vi "recunoastere_interfete_v2.vi"() -> (0 "Oscilloscope":string[](array[string]), 1 "DMM":string[](array[string]), 2 "Electronic Load":string[](array[string]), 3 "Source":string[](array[string]), 4 "Climate Chamber":string[](array[string]))   [LabVIEW 2022 SP3]
uses:
  <vilib>/regexp/Match Regular Expression.xnode
panel:
  out "Climate Chamber":i32
  out "Osciloscope":i32
  out "EL":i32
  out "DMM":i32
  out "Source":i32
  out "Aparatura":string[](array[string])=["TOELLNER", "AGILENT", "B&K", "LECROY", "VOTSCH"]
  out "error out":errorcluster
  in  "Instruments":string[](array[string])
  out "find list":string[](array[string])
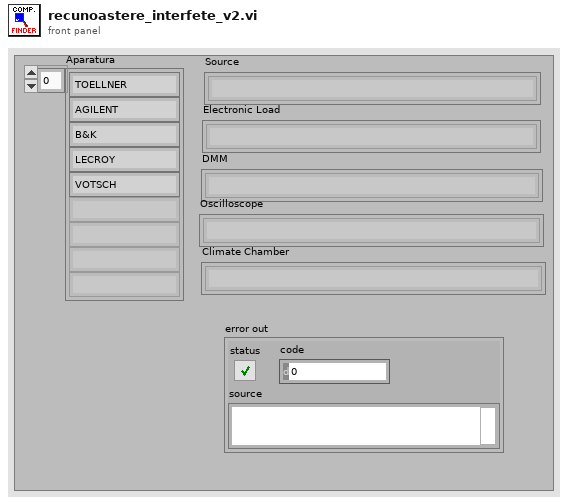
[diagram p1: front panel]
types:
  T1 = cluster{"Interface":u16, i32, "GPIB Device":u8, "GPIB Board":u8, "Direct Interface":bool, "String":string}
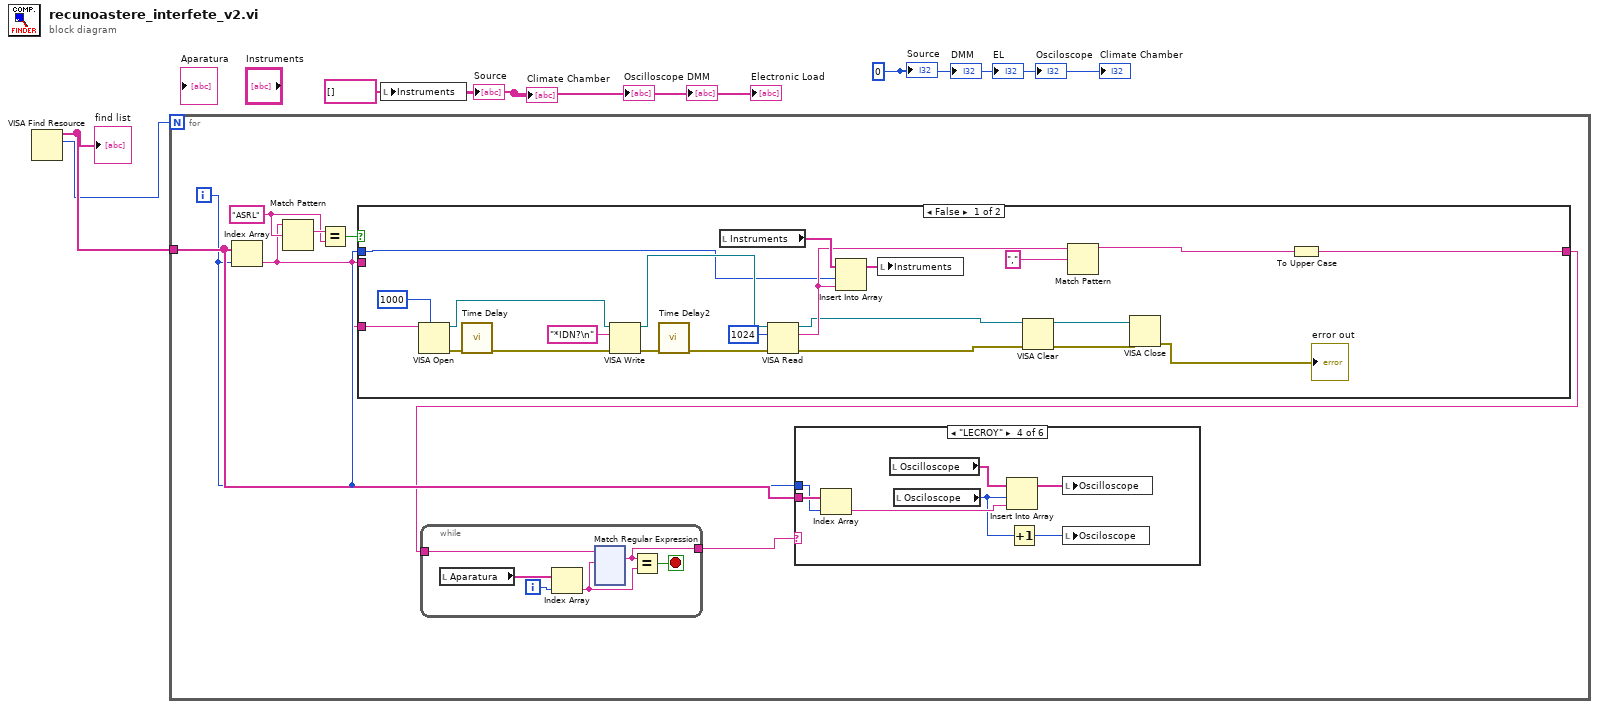
[diagram p0: block diagram]
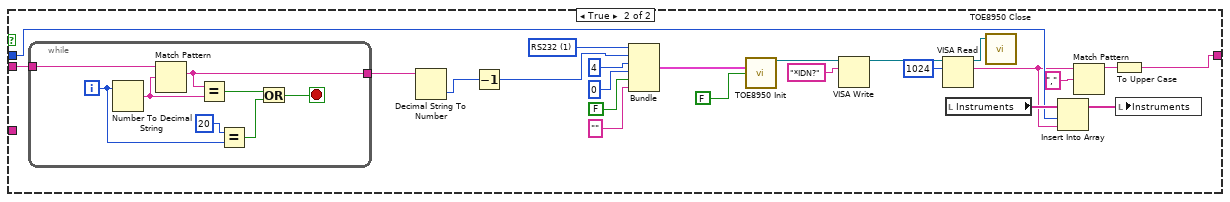
[diagram p2: hidden frame]
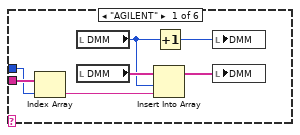
[diagram p3: hidden frame]
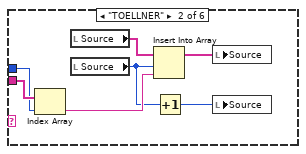
[diagram p4: hidden frame]
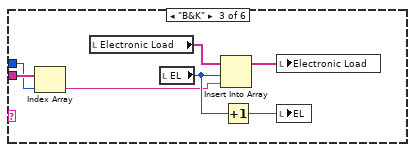
[diagram p5: hidden frame]
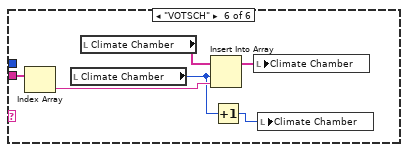
[diagram p7: hidden frame]
diagram:
  w3 = 0 ("Numeric")
  w4 = string[] [] ("Array")
  n1 = VISA Find Resource() -> (2:w1:u32, 3:w2:string[])  [unwired: 3 in, 1 out]
  "find list" <- w2
  n2 = for {
    N: w1 -> [_]
    tunnel: w2 -> [w12]
    i -> [w9]
    w7 = "ASRL" ("regular expression")
    n3 = Index Array(array=w12, index=w9) -> (element=w5:string)
    n4 = Match Pattern(string=w5, regular expression=w7) -> (match substring=w8:string)  [unwired: 1 in, 3 out]
    n5 = Equal?(x=w8, y=w7) -> (x = y?=w6:bool)
    n6 = case shown="False" w6 {
      tunnel: [w21 w39] -> w11
      tunnel: w9 -> [w20 w44]
      tunnel: w5 -> [w19 _]
      tunnel: w5 -> [_ w57]
      frame False {
        n7 = VISA Open(timeout (0)=u32 1000 ("VISA Open timeout (0)"), VISA resource name=w19) -> (VISA resource name=w29:refnum<visa-resource-name>, error out=w27:errorcluster)  [unwired: 3 in]
        n8 = call "Time Delay"("error in (no error)"=w27) -> ("error out"=w28:errorcluster)  [unwired: 10 in]
        n9 = VISA Write(VISA resource name=w29, write buffer="*IDN?\n", error in (no error)=w28) -> (VISA resource name out=w30:refnum<visa-resource-name>, error out=w26:errorcluster)  [unwired: 1 out]
        n10 = call "Time Delay2"("error in (no error)"=w26) -> ("error out"=w25:errorcluster)  [unwired: 10 in]
        n11 = local read "Instruments"() -> (w32:string[])
        n12 = VISA Read(VISA resource name=w30, byte count=u32 1024, error in (no error)=w25) -> (VISA resource name out=w17:refnum<visa-resource-name>, read buffer=w24:string, error out=w16:errorcluster)  [unwired: 1 out]
        n13 = Insert Into Array(array=w32, index=w20, new element=w24) -> (w31:string[])
        n14 = local write "Instruments"(w31) -> ()
        n15 = VISA Clear(VISA resource name=w17, error in (no error)=w16) -> (VISA resource name out=w14:refnum<visa-resource-name>, error out=w15:errorcluster)
        n16 = Match Pattern(string=w24, regular expression=",") -> (before substring=w22:string)  [unwired: 1 in, 3 out]
        n17 = VISA Close(VISA resource name=w14, error in (no error)=w15) -> (error out=→"error out":errorcluster)
        n18 = To Upper Case(1:w22) -> (0:w21:string)
      }
      frame True {
        w55 = u16 1 items=["GPIB", "RS232"] ("Interface")
        n19 = while {
          tunnel: w57 -> [w65]
          tunnel: [w58] -> w56
          i -> [w62]
          stop <- w59 stop-if-true
          n20 = Number To Decimal String(number=w62) -> (decimal integer string=w64:string)  [unwired: 1 in]
          n21 = Match Pattern(string=w65, regular expression=w64) -> (match substring=w58:string)  [unwired: 1 in, 3 out]
          n22 = Equal?(x=w58, y=w64) -> (x = y?=w63:bool)
          n23 = Equal?(x=20, y=w62) -> (x = y?=w60:bool)
          n24 = Or(x=w63, y=w60) -> (x .or. y?=w59:bool)
        }
        n25 = Decimal String To Number(string=w56) -> (number=w36:i32)  [unwired: 2 in, 1 out]
        n26 = Decrement(x=w36) -> (x-1=w35:i32)
        n27 = Bundle("Interface"=w55, w35, "GPIB Device"=u8 4, "GPIB Board"=u8 0, "Direct Interface"=FALSE, "String"="") -> (w50:T1)  [unwired: 1 in]
        n28 = call "TOE8950 Init.vi"("Select Interface"=w50, "Init Box Execute?"=FALSE) -> ("instr handle out"=w49:refnum<visa-resource-name>)  [unwired: 11 in, 2 out]
        n29 = VISA Write(VISA resource name=w49, write buffer="*IDN?") -> (VISA resource name out=w47:refnum<visa-resource-name>)  [unwired: 1 in, 2 out]
        n30 = VISA Read(VISA resource name=w47, byte count=u32 1024) -> (VISA resource name out=w43:refnum<visa-resource-name>, read buffer=w41:string)  [unwired: 1 in, 2 out]
        n31 = local read "Instruments"() -> (w46:string[])
        n32 = call "TOE8950 Close.vi"("instr handle in"=w43) -> ()  [unwired: 5 in, 1 out]
        n33 = Insert Into Array(array=w46, index=w44, new element=w41) -> (w45:string[])
        n34 = Match Pattern(string=w41, regular expression=",") -> (before substring=w40:string)  [unwired: 1 in, 3 out]
        n35 = To Upper Case(1:w40) -> (0:w39:string)
        n36 = local write "Instruments"(w45) -> ()
      }
    }
    n37 = while {
      tunnel: w11 -> [w69]
      tunnel: [w67] -> w10
      i -> [w71]
      stop <- w70 stop-if-true
      n38 = local read "Aparatura"() -> (w66:string[])
      n39 = Index Array(array=w66, index=w71) -> (element=w68:string)
      n40 = xnode "Match Regular Expression"("input string"=w69, "regular expression"=w68) -> ("whole match"=w67:string)  [unwired: 4 in, 4 out]
      n41 = Equal?(x=w67, y=w68) -> (x = y?=w70:bool)
    }
    n42 = case shown="\"LECROY\"" w10 {
      tunnel: w9 -> [w194 w201 w208 w215 _ _]
      tunnel: w12 -> [w195 w202 w209 w216 _ w219]
      frame "AGILENT" {
        n43 = Index Array(array=w195, index=w194) -> (element=w189:string)
        n44 = local read "DMM"() -> (w190:i32)
        n45 = local read "DMM"() -> (w193:string[])
        n46 = Insert Into Array(array=w193, index=w190, new element=w189) -> (w192:string[])
        n47 = Increment(x=w190) -> (x+1=w191:i32)
        n48 = local write "DMM"(w191) -> ()
        n49 = local write "DMM"(w192) -> ()
      }
      frame "TOELLNER" {
        n50 = Index Array(array=w202, index=w201) -> (element=w200:string)
        n51 = local read "Source"() -> (w196:string[])
        n52 = local read "Source"() -> (w198:i32)
        n53 = Insert Into Array(array=w196, index=w198, new element=w200) -> (w199:string[])
        n54 = Increment(x=w198) -> (x+1=w197:i32)
        n55 = local write "Source"(w199) -> ()
        n56 = local write "Source"(w197) -> ()
      }
      frame "B&K" {
        n57 = Index Array(array=w209, index=w208) -> (element=w203:string)
        n58 = local read "Electronic Load"() -> (w207:string[])
        n59 = local read "EL"() -> (w205:i32)
        n60 = Insert Into Array(array=w207, index=w205, new element=w203) -> (w206:string[])
        n61 = Increment(x=w205) -> (x+1=w204:i32)
        n62 = local write "Electronic Load"(w206) -> ()
        n63 = local write "EL"(w204) -> ()
      }
      frame "LECROY" {
        n64 = Index Array(array=w216, index=w215) -> (element=w212:string)
        n65 = local read "Oscilloscope"() -> (w214:string[])
        n66 = local read "Osciloscope"() -> (w211:i32)
        n67 = Insert Into Array(array=w214, index=w211, new element=w212) -> (w213:string[])
        n68 = Increment(x=w211) -> (x+1=w210:i32)
        n69 = local write "Oscilloscope"(w213) -> ()
        n70 = local write "Osciloscope"(w210) -> ()
      }
      frame "False", Default {
      }
      frame "VOTSCH" {
        n71 = Index Array(array=w219) -> (element=w220:string)  [unwired: 1 in]
        n72 = local read "Climate Chamber"() -> (w218:i32)
        n73 = local read "Climate Chamber"() -> (w222:string[])
        n74 = Insert Into Array(array=w222, index=w218, new element=w220) -> (w221:string[])
        n75 = Increment(x=w218) -> (x+1=w217:i32)
        n76 = local write "Climate Chamber"(w221) -> ()
        n77 = local write "Climate Chamber"(w217) -> ()
      }
    }
  }
  n78 = local write "Instruments"(w4) -> ()
  "Source" <- w4
  "Electronic Load" <- w4
  "Oscilloscope" <- w4
  "DMM" <- w4
  "Source" <- w3
  "DMM" <- w3
  "EL" <- w3
  "Osciloscope" <- w3
  "Climate Chamber" <- w4
  "Climate Chamber" <- w3
